vi "6000_watchdog_ticker.vi"() -> ()   [LabVIEW 2010]
panel:
  in  "Port Name":string
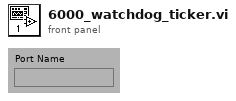
[diagram p1: front panel]
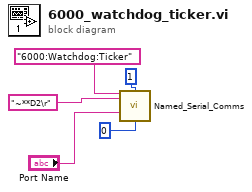
[diagram p0: block diagram]
diagram:
  n1 = call "Named_Serial_Comms.vi"("Channel Name"="6000:Watchdog:Ticker", "Write String"="~**D2\r", "Timeout/ms"=u32 1, "Port Name"="Port Name", "Terminate Count"=i16 0 ("!Terminate Count")) -> ()  [unwired: 7 in, 4 out]
